vi "PRIME Detector Format CONFIG command with offsets.vi"(11 "Offsets":u16[][](array[numeric])=[[0, 0, 0, 0, 0, 0, 0, 0, 0, 0, 0, 0, 0, 0, 0, 0, 0, 0, 0, 0, 0, 0, 0, 0, 0, 0, 0, 0, 0, 0, 0, 0]] format="%04x") -> (3 "Command":string)   [LabVIEW 2024, in "PRIME Detector.lvclass"]
uses:
  PRIME Detector.lvclass
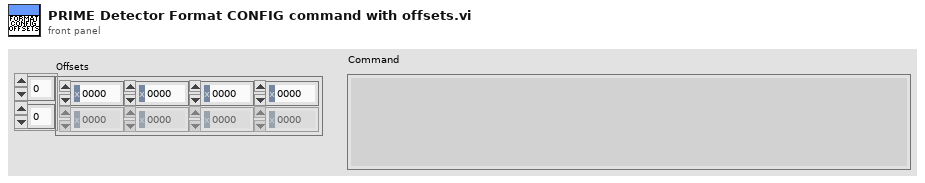
[diagram p1: front panel]
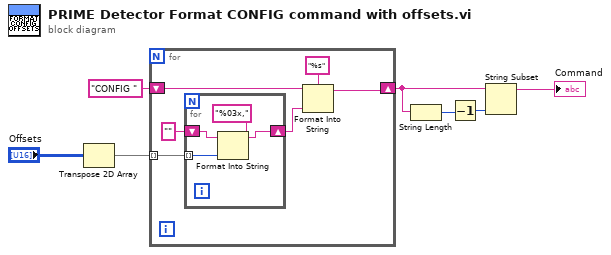
[diagram p0: block diagram]
diagram:
  n1 = Transpose 2D Array(2D array="Offsets") -> (transposed array=w1:u16[][])
  n2 = for {
    tunnel: w1 -> [w10] mode=indexing
    shift-right: [w11] -> w4
    shift-left: "CONFIG " ("Command") -> [w13]
    n3 = for {
      tunnel: w10 -> [w16] mode=indexing
      shift-right: [w14] -> w8
      shift-left: "" -> [w15]
      n4 = Format Into String(format string="%03x,", initial string=w15, w16) -> (resulting string=w14:string)  [unwired: 1 in, 1 out]
    }
    n5 = Format Into String(format string="%s", initial string=w13, w8) -> (resulting string=w11:string)  [unwired: 1 in, 1 out]
  }
  n6 = String Length(string=w4) -> (length=w3:i32)
  n7 = Decrement(x=w3) -> (x-1=w2:i32)
  n8 = String Subset(string=w4, length (rest)=w2) -> (substring=→"Command":string)  [unwired: 1 in]
